vi "EOD Read.vi"(8 "error in (no error)":errorcluster, 11 "Path":path) -> (0 "error out":errorcluster, 1 "EODDataOut":T1(array[cluster]), 2 "Iteration Number":i32)   [LabVIEW 2014]
panel:
  out "Wave Offset":i32[](array[numeric])
  # "EOD File Reader VI"
  # "Inputs"
  # "Outputs"
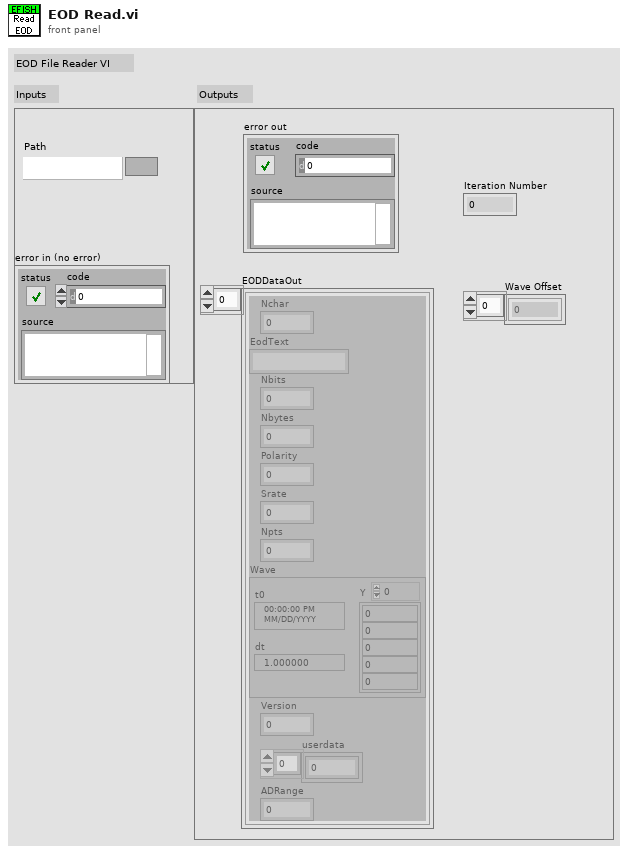
[diagram p1: front panel]
types:
  T1 = cluster{"Nchar":i32, "EodText":string, "Nbits":i32, "Nbytes":i32, "Polarity":i32, "Srate":i32, "Npts":i32, "Wave":waveform(dbl), "Version":i32, "userdata":dbl[], "ADRange":dbl}[]
  T2 = enum16{"open", "replace", "create", "open or create", "replace or create", "replace or create with confirmation"}
  T3 = cluster{u8, string, i8, i8, i8, u32, u32, "Waveform":waveform(i16), "Version":i32, sgl[], sgl}
  T4 = cluster{"Nchar":i32, "EodText":string, "Nbits":i32, "Nbytes":i32, "Polarity":i32, "Srate":u32, "Npts":u32, "Wave":waveform(dbl), "Version":i32, "userdata":dbl[], "ADRange":dbl}[]
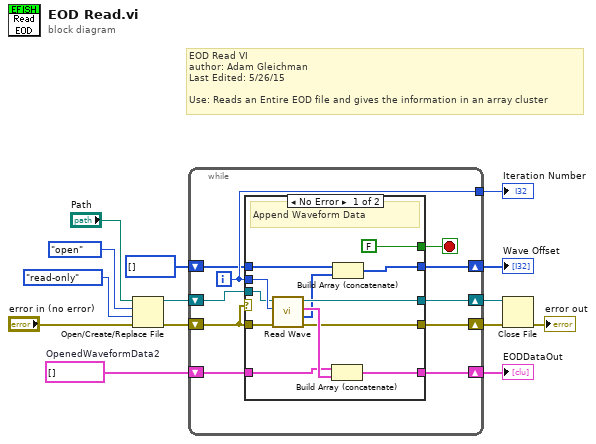
[diagram p0: block diagram]
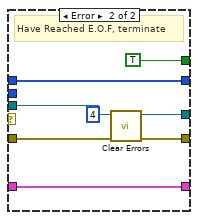
[diagram p2: hidden frame]
diagram:
  w14 = T1 []  # OpenedWaveformData2
  # "EOD Read VI\nauthor: Adam Gleichman\nLast Edited: 5/26/15\n\nUse: Reads an Entire EOD file and gives the information in an array cluster"
  n1 = Open/Create/Replace File(file path (use dialog)="Path", error in="error in (no error)", operation (0:open)=T2."open", access (0:read/write)=enum16{"read/write", "read-only", "write-only"}."read-only") -> (refnum out=w8:refnum<file>, error out=w4:errorcluster)  [unwired: 2 in, 1 out]
  n2 = while {
    shift-right: [w21] -> w3
    shift-left: w8 -> [w24]
    shift-right: [w20] -> w2
    shift-left: w4 -> [w18]
    shift-right: [w22] -> w13
    shift-left: w14 -> [w23]
    tunnel: [w19] -> w12
    shift-right: [w15] -> w10
    shift-left: i32[] [] -> [w16]
    i -> [w19]
    stop <- w17 stop-if-true
    n3 = case shown="No Error" w18 {
      tunnel: w19 -> [w36 _]
      tunnel: w18 -> [w35 w38]
      tunnel: w24 -> [w34 w42]
      tunnel: w23 -> [w31 w43]
      tunnel: [w32 w43] -> w22
      tunnel: [w30 w42] -> w21
      tunnel: [w29 w37] -> w20
      tunnel: [FALSE TRUE] -> w17
      tunnel: w16 -> [w27 w40]
      tunnel: [w25 w40] -> w15
      frame No Error {
        # "Append Waveform Data"
        n4 = call "Read Wave.vi"("error in"=w35, "Iteration of Loop"=w36, "refnum"=w34) -> ("error out"=w29:errorcluster, "Wave Offset"=w26:i32[], "output cluster"=w33:T3, "refnum out"=w30:refnum<file>)  [unwired: 4 in]
        n5 = Build Array (concatenate)(w31, w33) -> (w32:T4)
        n6 = Build Array (concatenate)(w27, w26) -> (w25:i32[])
      }
      frame Error {
        # "Have Reached E.O.F, terminate"
        n7 = call <vilib>:"Clear Errors.vi"("error in (no error)"=w38, "specific error code to clear (0: all)"=4) -> ("error out"=w37:errorcluster)  [unwired: 4 in, 1 out]
      }
    }
  }
  "Iteration Number" <- w12
  "Wave Offset" <- w10
  "EODDataOut" <- w13
  n8 = Close File(refnum=w3, error in=w2) -> (error out=→"error out":errorcluster)  [unwired: 1 out]
